vi "Read Continuous.vi"(8 "error in (no error)":errorcluster, 11 "Data Source in":refnum<class "Data Source.lvclass">) -> (0 "error out":errorcluster, 2 "Continuous":bool, 3 "Data Source out":refnum<class "Data Source.lvclass">)   [LabVIEW 2020, in "Data Source.lvlib" / "Data Source.lvclass"]
uses:
  Data Source.lvclass
  Data Source.lvclass/Data Source.ctl
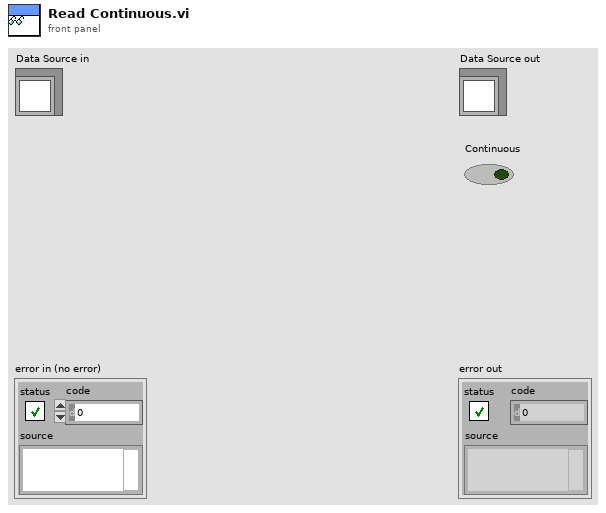
[diagram p1: front panel]
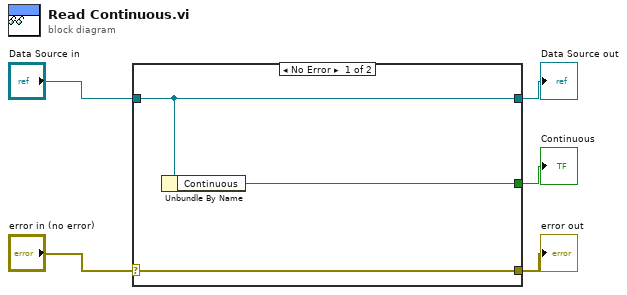
[diagram p0: block diagram]
diagram:
  n1 = case shown="No Error" "error in (no error)" {
    selector: "error in (no error)" -> [w8 w9]
    tunnel: [w8 w9] -> w4
    tunnel: [w7 w10] -> w2
    tunnel: "Data Source in" -> [w7 w10]
    tunnel: [w6 _] -> w1
    frame No Error {
      n2 = Unbundle By Name(w7) -> ("Continuous"=w6:bool)
    }
    frame Error {
    }
  }
  "error out" <- w4
  "Data Source out" <- w2
  "Continuous" <- w1
